vi "Read.vi"(8 "error in (no error)":errorcluster, 10 "# Samples to read":i32=1000000, 11 "device handle in":T1) -> (0 "error out":errorcluster, 1 "Actual # Samples":i32, 2 "Samples":u8[](array[numeric]), 3 "device handle out":T1)   [LabVIEW 2023, in "RTL-SDR.lvlib"]
uses:
  RTL-SDR.lvlib
  Controls/Device Handle.ctl
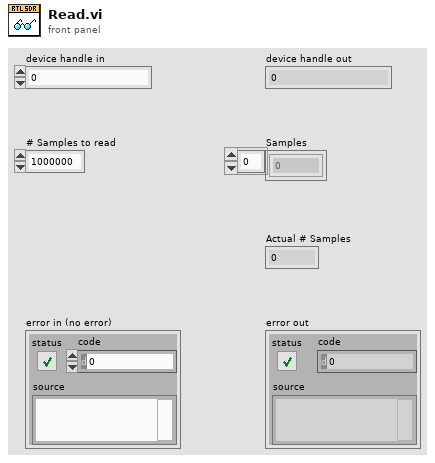
[diagram p1: front panel]
types:
  T1 = typedef "RTL-SDR.lvlib/Device Handle.ctl" = u64
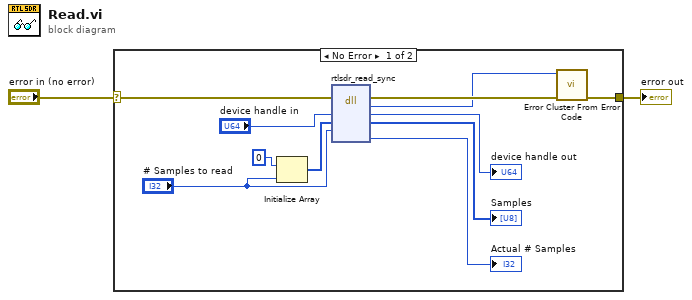
[diagram p0: block diagram]
diagram:
  n1 = case shown="No Error" "error in (no error)" {
    selector: "error in (no error)" -> [w10 w14]
    tunnel: [w4 w14] -> w2
    frame No Error {
      n2 = Initialize Array(u8 0, "# Samples to read") -> (w7:u8[])
      n3 = dll-call lib="usr/local/Cellar/librtlsdr/0.6.0/bin/rtl_sdr" fn="rtlsdr_read_sync"(error in=w10, "dev"="device handle in", "buf"=w7, "len"="# Samples to read") -> (error out=w13:errorcluster, "return type"=w3:i32, "dev"=→"device handle out":u64, "buf"=→"Samples":u8[], "n_read"=→"Actual # Samples":i32)  [unwired: 4 in, 1 out]
      n4 = call <vilib>:"Error Cluster From Error Code.vi"("error in (no error)"=w13, "error code (0)"=w3) -> ("error out"=w4:errorcluster)  [unwired: 7 in]
    }
    frame Error {
    }
  }
  "error out" <- w2
